vi "CANtest.vi"() -> ()   [LabVIEW 2017]
uses:
  <vilib>/addons/Maxon Motor/EPOS2 CANopen/CANopen/sbCANopenBaseClass.lvclass
  <vilib>/Platform/TimedLoop/XDataNode/timing_clust.ctl
  <vilib>/Platform/TimedLoop/XDataNode/nitl_modes.ctl
  <vilib>/Platform/TimedLoop/XDataNode/wakeup.ctl
  <vilib>/Platform/TimedLoop/XDataNode/XDataNode.xnode
  <vilib>/Platform/TimedLoop/XDataNode/XDNodeRunTimeDep.lvlib
panel:
  in  "motor enable":i32
  in  "enable ready 2":bool
  out "Finished Late? [i-1] 3":bool
  out "Numeric 3":i32
  out "Iteration Duration 2":i64
  out "Finished Late? [i-1]":bool
  out "Node ID\nin while loop 2":u8
  out "Node ID\nin while loop":u8
  out "Array":refnum<class "sbCANopenBaseClass.lvclass">[](array[class])
  out "for 1":i32
  out "while loop":i32
  in  "Loop 2":bool
  in  "Current":i32=10
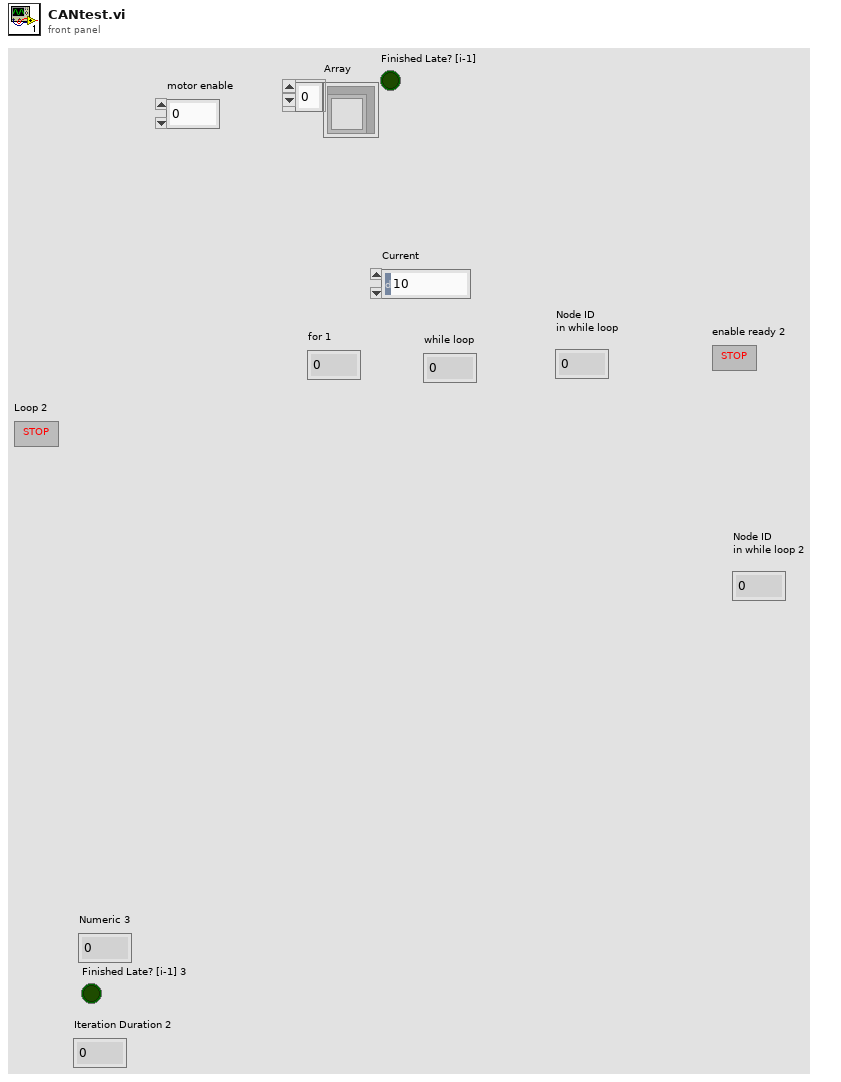
[diagram p1: front panel]
types:
  T1 = typedef "XDNodeRunTimeDep.lvlib/timing_clust.ctl" = cluster{"Expected End [f-1]":u64, "Actual End [f-1]":u64, "Finished Late? [f-1]":bool, "Expected End [i-1]":u64, "Actual End [i-1]":u64, "Finished Late? [i-1]":bool, "Expected Start [i]":u64, "Actual Start [i]":u64, "Expected Start [f]":u64, "Actual Start [f]":u64, "Source Name":string, "Structure Name":string, "Period":i64, "Deadline":i64, "Offset":i64, "Start":i64, "Priority":i32, "Timeout":i32, "Mode":T2, "Wakeup Reason":T3, "Error":errorcluster, "Source Type":string, "Secondary Source Type":string, "Global End Time":u64, "Global Start Time":u64, "Frame Duration":u64, "Iteration Duration":u64, "Assigned CPU":i32, "I/O Scan Engine Mode":u32}
  T2 = typedef "XDNodeRunTimeDep.lvlib/nitl_modes.ctl" = enum32{"No Change", "Process missed periods, maintain original phase", "Discard missed periods, maintain original phase", "Process missed periods, ignore original phase", "Discard missed periods, ignore original phase"}
  T3 = typedef "XDNodeRunTimeDep.lvlib/wakeup.ctl" = enum32{"Normal", "Aborted", "Asynchronous wakeup", "Timing source error", "Timed loop error", "Timeout"}
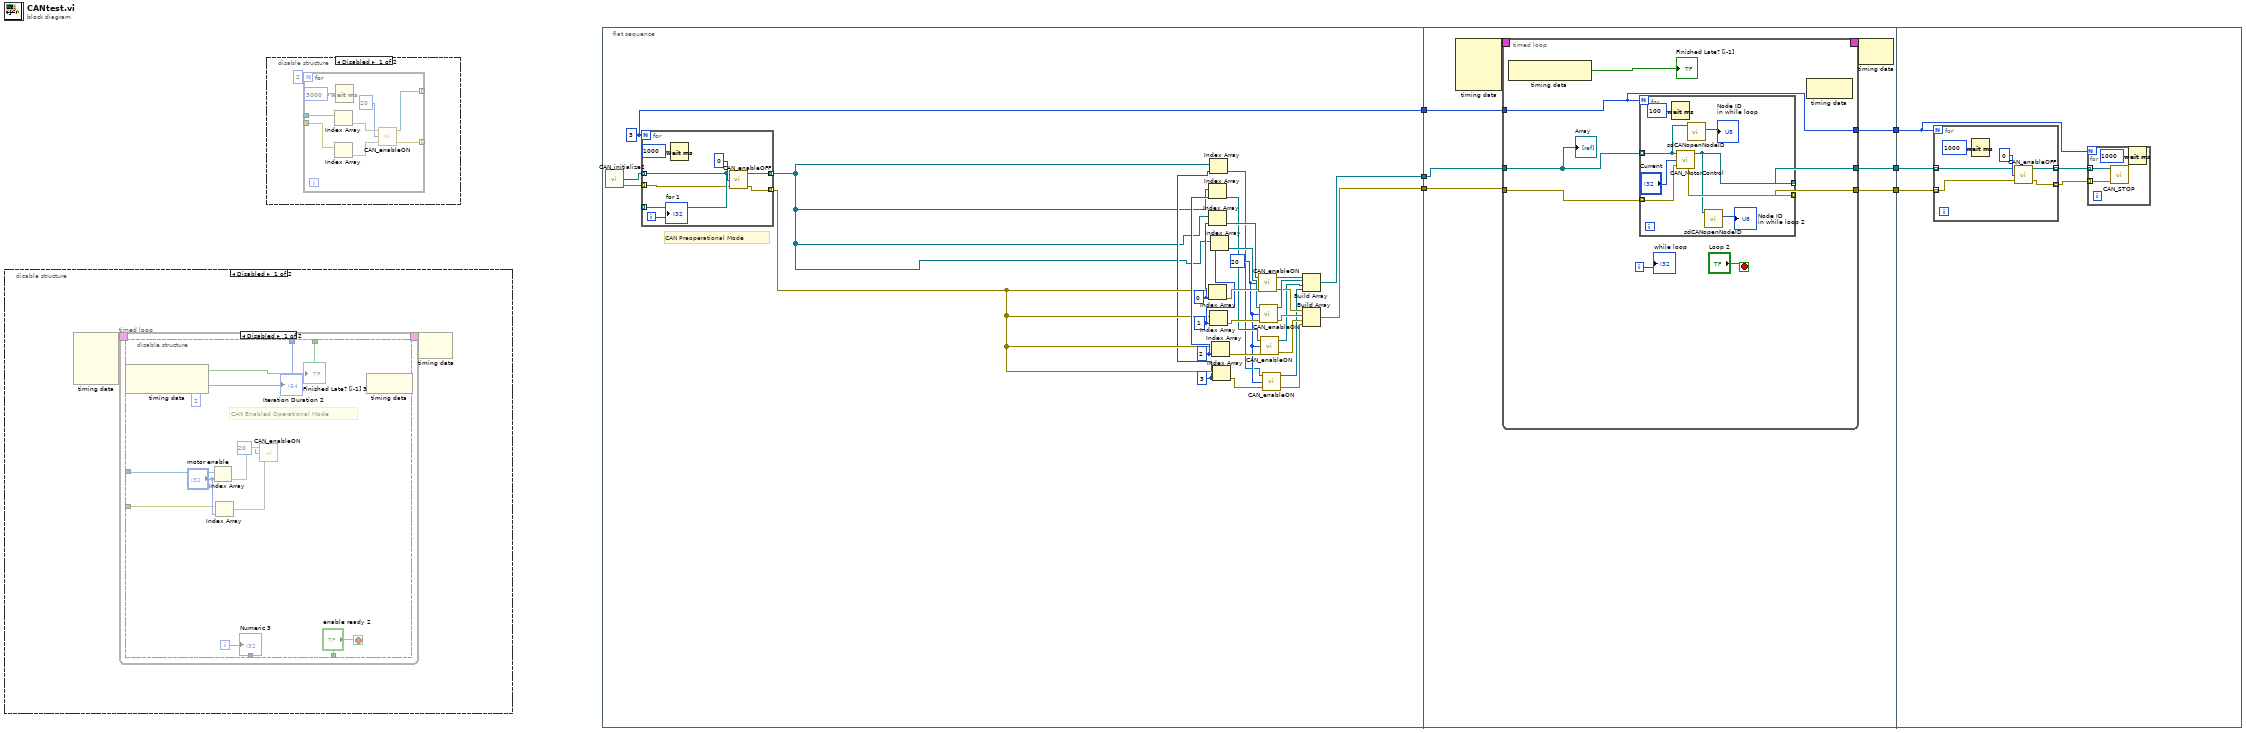
[diagram p0: block diagram]
diagram:
  n1 = disable-structure shown="Disabled" {
    frame Disabled {
      n2 = node-c288() -> (w8:T1)  [unwired: 4 in]
      n3 = timed-loop {
        timing: w8 -> [_]
        timing-out: [_] -> w7
        i -> [w10]
        stop <- w12 stop-if-true
        n4 = node-c288() -> (w11:bool, w9:i64)  [unwired: 1 in]
        n5 = disable-structure shown="Disabled" {
          disable-tunnel: ["enable ready 2" _] -> w12
          disable-tunnel: w11 -> [w21 _]
          disable-tunnel: w10 -> [w20 _]
          disable-tunnel: w9 -> [w19 _]
          disable-tunnel: _ -> [w16 _]
          disable-tunnel: _ -> [w14 _]
          frame Disabled {
            (unwired) 2
            # "CAN Enabled Operational Mode"
            n6 = Index Array(array=w16, index="motor enable") -> (element=w18)
            n7 = Index Array(array=w14, index="motor enable") -> (element=w17)
            n8 = call "CAN_enableON.vi"("error in (no error)"=w17, "Current"=20, "sbCANopenBaseClass in"=w18) -> ()  [unwired: 1 in, 2 out]
            "Finished Late? [i-1] 3" <- w21
            "Numeric 3" <- w20
            "Iteration Duration 2" <- w19
          }
          frame Enabled {
          }
        }
        n9 = node-c288() -> ()  [unwired: 1 in, 1 out]
      }
      n10 = node-c288(w7) -> ()  [unwired: 1 out]
    }
    frame Enabled {
    }
  }
  n11 = disable-structure shown="Disabled" {
    frame Disabled {
      n12 = for {
        N: 2 -> [_]
        tunnel: _ -> [w37]
        tunnel: _ -> [w35]
        tunnel: [w32] -> _ mode=indexing
        tunnel: [w31] -> _ mode=indexing
        n13 = Index Array(array=w35) -> (element=w34)  [unwired: 1 in]
        n14 = Index Array(array=w37) -> (element=w36)  [unwired: 1 in]
        n15 = Wait (ms)(milliseconds to wait=u32 3000) -> ()  [unwired: 1 out]
        n16 = call "CAN_enableON.vi"("error in (no error)"=w34, "Current"=20, "sbCANopenBaseClass in"=w36) -> ("error out"=w31:errorcluster, "CANopen Session Out"=w32:refnum<class "sbCANopenBaseClass.lvclass">)  [unwired: 1 in]
      }
    }
    frame Enabled {
    }
  }
  n17 = flat-sequence {
    tunnel: [w64] -> w4
    tunnel: [w65] -> w3
    tunnel: [w40] -> w2
    tunnel: [w78] -> w6
    tunnel: [w77] -> w5
    tunnel: w4 -> [w80]
    tunnel: w3 -> [w79]
    tunnel: w2 -> [w74]
    tunnel: [w73] -> w1
    tunnel: w6 -> [w104]
    tunnel: w5 -> [w103]
    tunnel: w1 -> [w102]
    frame #0 {
      w40 = 3
      w46 = 3 ("index")
      w53 = 2 ("index")
      w55 = 1 ("index")
      w63 = 0 ("index")
      w45 = 20 ("Current")
      # "CAN Preoperational Mode"
      n18 = call "CAN_initialize2.vi"() -> ("Array 2"=w38:errorcluster[], "Array"=w39:refnum<class "sbCANopenBaseClass.lvclass">[])  [unwired: 3 in, 1 out]
      n19 = for {
        N: w40 -> [_]
        tunnel: [w70] -> _ mode=indexing
        tunnel: [w71] -> w48 mode=indexing
        tunnel: w39 -> [w70] mode=indexing
        tunnel: w38 -> [w69] mode=indexing
        tunnel: [w66] -> w44 mode=indexing
        i -> [w67]
        n20 = Wait (ms)(milliseconds to wait=u32 1000) -> ()  [unwired: 1 out]
        n21 = call "CAN_enableOFF.vi"("error in (no error)"=w69, "Current"=0, "sbCANopenBaseClass in"=w70) -> ("error out"=w71:errorcluster, "CANopen Session Out"=w66:refnum<class "sbCANopenBaseClass.lvclass">)  [unwired: 1 in]
        "for 1" <- w67
      }
      n22 = Index Array(array=w44, index=w63) -> (element=w56:refnum<class "sbCANopenBaseClass.lvclass">)
      n23 = Index Array(array=w44, index=w53) -> (element=w52:refnum<class "sbCANopenBaseClass.lvclass">)
      n24 = Index Array(array=w48, index=w63) -> (element=w59:errorcluster)
      n25 = Index Array(array=w44, index=w46) -> (element=w43:refnum<class "sbCANopenBaseClass.lvclass">)
      n26 = Index Array(array=w48, index=w55) -> (element=w60:errorcluster)
      n27 = Index Array(array=w44, index=w55) -> (element=w54:refnum<class "sbCANopenBaseClass.lvclass">)
      n28 = Index Array(array=w48, index=w53) -> (element=w51:errorcluster)
      n29 = Index Array(array=w48, index=w46) -> (element=w47:errorcluster)
      n30 = call "CAN_enableON.vi"("error in (no error)"=w59, "Current"=w45, "sbCANopenBaseClass in"=w56) -> ("error out"=w58:errorcluster, "CANopen Session Out"=w62:refnum<class "sbCANopenBaseClass.lvclass">)  [unwired: 1 in]
      n31 = call "CAN_enableON.vi"("error in (no error)"=w60, "Current"=w45, "sbCANopenBaseClass in"=w54) -> ("error out"=w57:errorcluster, "CANopen Session Out"=w61:refnum<class "sbCANopenBaseClass.lvclass">)  [unwired: 1 in]
      n32 = call "CAN_enableON.vi"("error in (no error)"=w51, "Current"=w45, "sbCANopenBaseClass in"=w52) -> ("error out"=w49:errorcluster, "CANopen Session Out"=w50:refnum<class "sbCANopenBaseClass.lvclass">)  [unwired: 1 in]
      n33 = call "CAN_enableON.vi"("error in (no error)"=w47, "Current"=w45, "sbCANopenBaseClass in"=w43) -> ("error out"=w41:errorcluster, "CANopen Session Out"=w42:refnum<class "sbCANopenBaseClass.lvclass">)  [unwired: 1 in]
      n34 = Build Array(w62, w61, w50, w42) -> (w64:refnum<class "sbCANopenBaseClass.lvclass">[])
      n35 = Build Array(w58, w57, w49, w41) -> (w65:errorcluster[])
    }
    frame #1 {
      n36 = node-c288() -> (w76:T1)  [unwired: 4 in]
      n37 = timed-loop {
        tunnel: w80 -> [w83]
        tunnel: [w86] -> w78
        tunnel: w79 -> [w82]
        tunnel: [w85] -> w77
        timing: w76 -> [_]
        timing-out: [_] -> w75
        tunnel: w74 -> [w81]
        tunnel: [w81] -> w73
        i -> [w87]
        stop <- "Loop 2" stop-if-true
        n38 = node-c288() -> (→"Finished Late? [i-1]":bool)  [unwired: 1 in]
        n39 = for {
          N: w81 -> [_]
          tunnel: [w93] -> w86 mode=indexing
          tunnel: [w99] -> w85 mode=indexing
          tunnel: w83 -> [w95] mode=indexing
          tunnel: w82 -> [w97] mode=indexing
          n40 = Wait (ms)(milliseconds to wait=u32 100) -> ()  [unwired: 1 out]
          n41 = call "CAN_MotorControl.vi"("sbCANopenBaseClass in"=w95, "Current"="Current", "error in (no error)"=w97) -> ("CANopen Session Out"=w93:refnum<class "sbCANopenBaseClass.lvclass">, "error out"=w99:errorcluster)  [unwired: 3 out]
          n42 = call-dynamic "sdCANopenNodeID.vi"("sbCANopenBaseClass in"=w95) -> ("Node ID"=→"Node ID\nin while loop":u8)  [unwired: 9 in, 1 out]
          n43 = call-dynamic "sdCANopenNodeID.vi"("sbCANopenBaseClass in"=w93) -> ("Node ID"=→"Node ID\nin while loop 2":u8)  [unwired: 9 in, 1 out]
        }
        n44 = node-c288() -> ()  [unwired: 1 in, 1 out]
        "while loop" <- w87
        "Array" <- w83
      }
      n45 = node-c288(w75) -> ()  [unwired: 1 out]
    }
    frame #2 {
      n46 = for {
        N: w102 -> [_]
        tunnel: [w115] -> w105 mode=indexing
        tunnel: [w113] -> w106 mode=indexing
        tunnel: w104 -> [w111] mode=indexing
        tunnel: w103 -> [w110] mode=indexing
        n47 = Wait (ms)(milliseconds to wait=u32 1000) -> ()  [unwired: 1 out]
        n48 = call "CAN_enableOFF.vi"("error in (no error)"=w110, "Current"=0, "sbCANopenBaseClass in"=w111) -> ("error out"=w113:errorcluster, "CANopen Session Out"=w115:refnum<class "sbCANopenBaseClass.lvclass">)  [unwired: 1 in]
      }
      n49 = for {
        N: w102 -> [_]
        tunnel: w105 -> [w109] mode=indexing
        tunnel: w106 -> [w108] mode=indexing
        n50 = call "CAN_STOP.vi"("error in"=w108, "CANopen Session In"=w109) -> ()  [unwired: 3 in, 1 out]
        n51 = Wait (ms)(milliseconds to wait=u32 1000) -> ()  [unwired: 1 out]
      }
    }
  }
